vi "SNTP Light Initialization VI.vi"(8 "error in (no error)":errorcluster, 10 "Custom XML":string, 11 "Device Item Ref in":T1 format="%.0x") -> (0 "error out":errorcluster, 3 "Device Item Ref out":T1 format="%.0x")   [LabVIEW 2013, in "SNTP Light Custom Device Configuration.lvlib"]
uses:
  SNTP Light Custom Device Configuration.lvlib
  <vilib>/NI Veristand/Custom Device API/Custom Device Item Ref.ctl
  <vilib>/NI Veristand/Custom Device API/Custom Device Channel.ctl
  <vilib>/NI Veristand/Custom Device API/Custom Device Channel Type.ctl
  <vilib>/NI Veristand/Custom Device API/Set Item Property (String).vi
  <vilib>/NI Veristand/Custom Device API/Set Item Property (U16).vi
  <vilib>/NI Veristand/Custom Device API/Set Item Property (Double).vi
  <vilib>/NI Veristand/Custom Device API/Set Item Property (Boolean).vi
  <vilib>/NI Veristand/Custom Device API/Custom Device API.lvlib
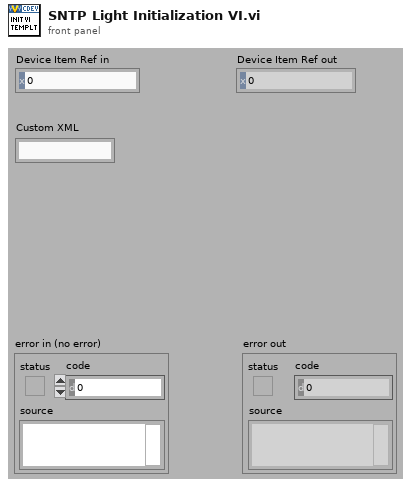
[diagram p1: front panel]
types:
  T1 = typedef "Custom Device API.lvlib/Custom Device Item Ref.ctl" = u64
  T2 = typedef "Custom Device API.lvlib/Custom Device Channel.ctl" = cluster{"Type":T3, "Units":string, "Default Value":dbl, "Faultable":bool, "Scalable":bool}
  T3 = typedef "Custom Device API.lvlib/Custom Device Channel Type.ctl" = enum16{"Input", "Output"}
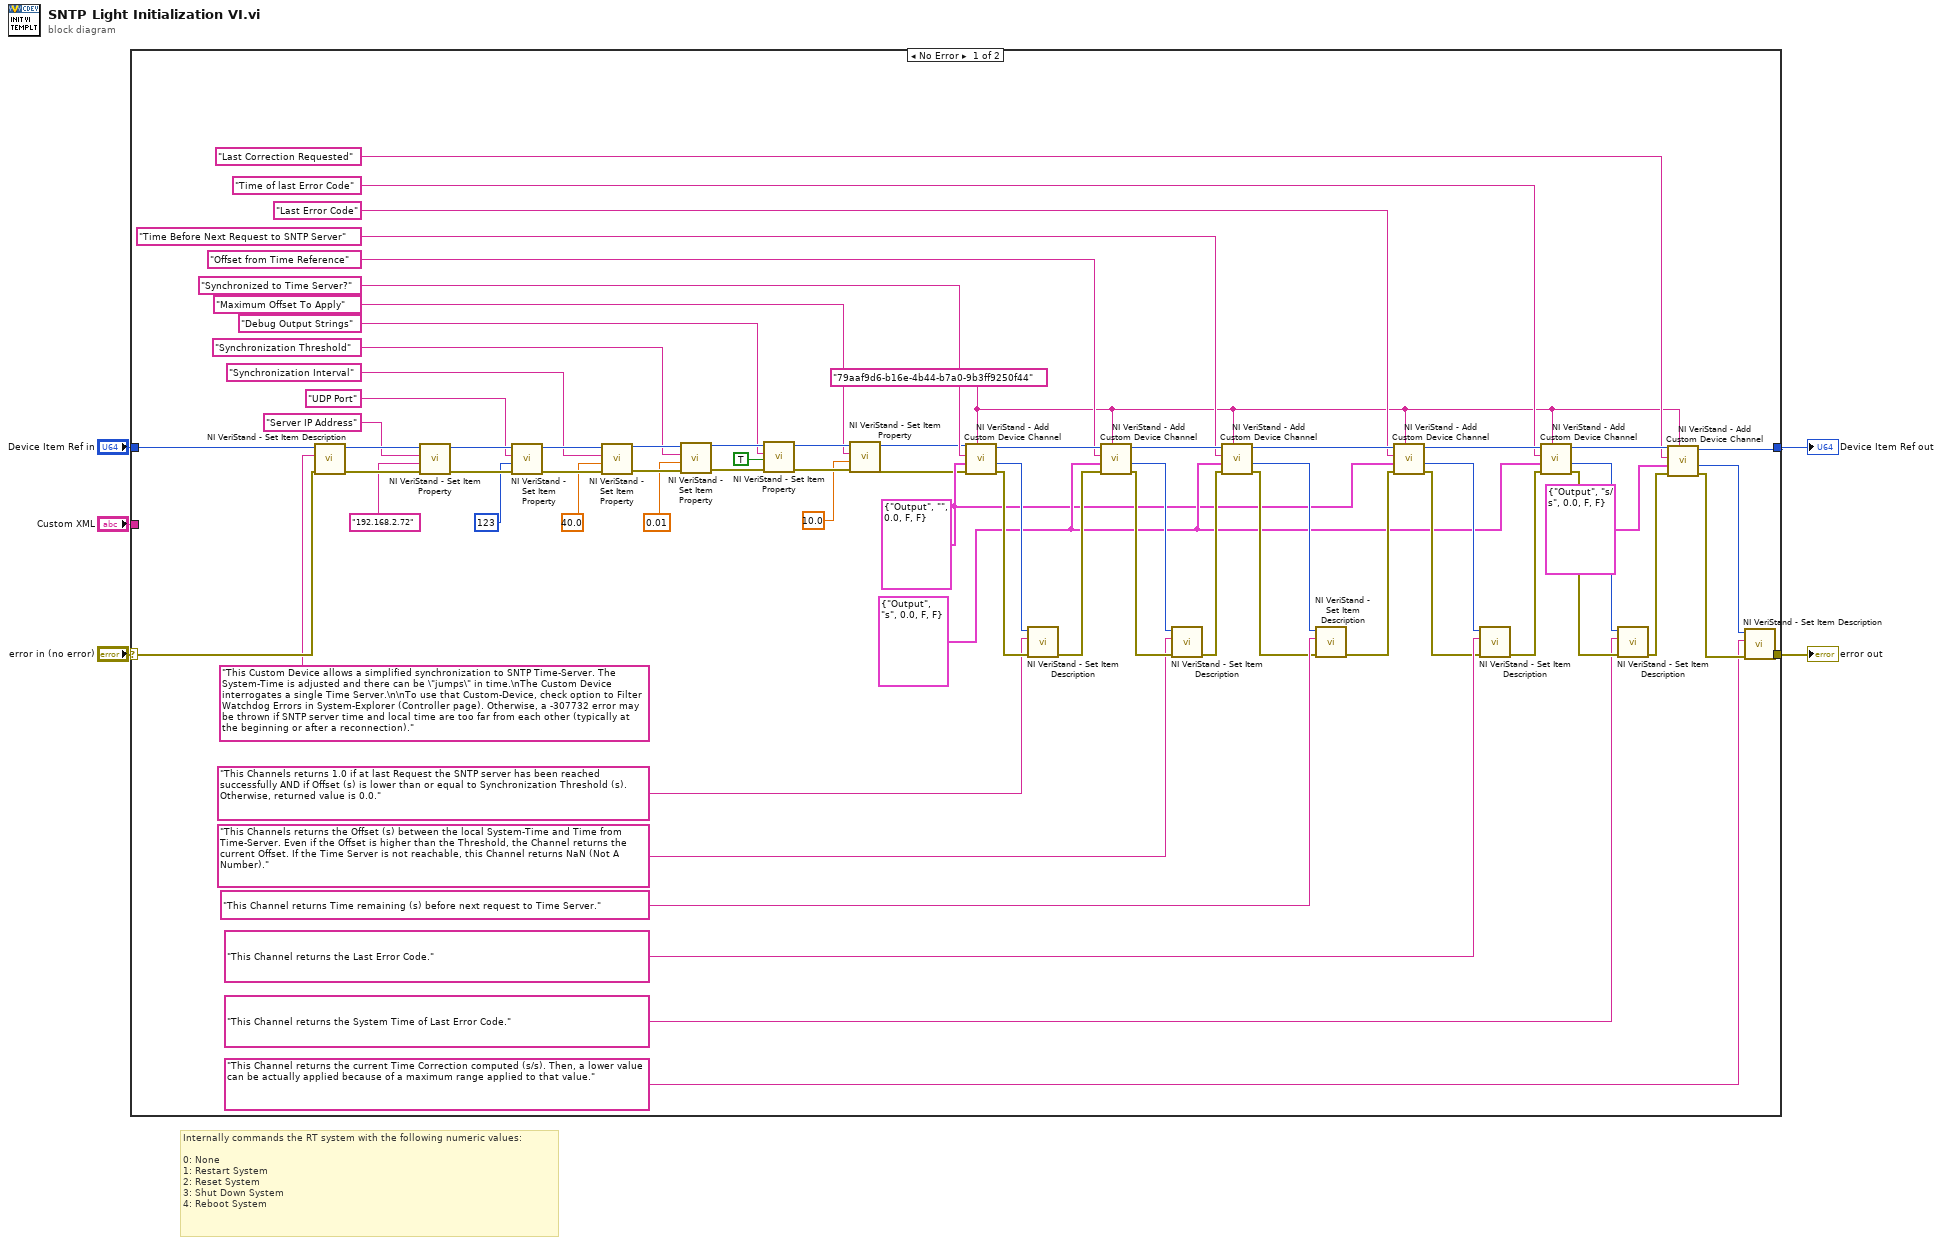
[diagram p0: block diagram]
diagram:
  # "Internally commands the RT system with the following numeric values:\n\n0: None\n1: Restart System\n2: Reset System\n3: Shut Down System\n4: Reboot System"
  n1 = case shown="No Error" "error in (no error)" {
    selector: "error in (no error)" -> [w73 w76]
    tunnel: [w6 w76] -> w5
    tunnel: [w7 w75] -> w3
    tunnel: "Device Item Ref in" -> [w74 w75]
    tunnel: "Custom XML" -> [_ _]
    frame No Error {
      w8 = "79aaf9d6-b16e-4b44-b7a0-9b3ff9250f44" ("GUID (Default Channel)")
      w19 = T2 {"Type"=enum."Output", "Units"="s", "Default Value"=0.0, "Faultable"=FALSE, "Scalable"=FALSE} ("Channel")
      w15 = T2 {"Type"=enum."Output", "Units"="", "Default Value"=0.0, "Faultable"=FALSE, "Scalable"=FALSE} ("Channel")
      n2 = call <vilib>:"NI VeriStand - Set Item Description.vi"("error in (no error)"=w73, "Description"="This Custom Device allows a simplified synchronization to SNTP Time-Server. The System-Time is adjusted and there can be \"jumps\" in time.\nThe Custom Device interrogates a single Time Server.\n\nTo use that Custom-Device, check option to Filter Watchdog Errors in System-Explorer (Controller page). Otherwise, a -307732 error may be thrown if SNTP server time and local time are too far from each other (typically at the beginning or after a reconnection).", "Item Ref in"=w74) -> ("error out"=w71:errorcluster, "Item Ref out"=w70:T1)  [unwired: 6 in, 1 out]
      n3 = call-poly <vilib>:"NI VeriStand - Set Item Property.vi"("error in (no error)"=w71, "Value"="192.168.2.72", "Property Name"="Server IP Address", "Item Ref in"=w70) -> ("error out"=w67:errorcluster, "Item Ref out"=w69:T1)  [unwired: 5 in, 1 out]
      n4 = call-poly <vilib>:"NI VeriStand - Set Item Property.vi"("error in (no error)"=w67, "Value"=u16 123, "Property Name"="UDP Port", "Item Ref in"=w69) -> ("error out"=w66:errorcluster, "Item Ref out"=w68:T1)  [unwired: 5 in, 1 out]
      n5 = call-poly <vilib>:"NI VeriStand - Set Item Property.vi"("error in (no error)"=w66, "Value"=40.0, "Property Name"="Synchronization Interval", "Item Ref in"=w68) -> ("error out"=w58:errorcluster, "Item Ref out"=w59:T1)  [unwired: 5 in, 1 out]
      n6 = call-poly <vilib>:"NI VeriStand - Set Item Property.vi"("error in (no error)"=w58, "Value"=0.01, "Property Name"="Synchronization Threshold", "Item Ref in"=w59) -> ("error out"=w30:errorcluster, "Item Ref out"=w31:T1)  [unwired: 5 in, 1 out]
      n7 = call-poly <vilib>:"NI VeriStand - Set Item Property.vi"("error in (no error)"=w30, "Value"=TRUE, "Property Name"="Debug Output Strings", "Item Ref in"=w31) -> ("error out"=w11:errorcluster, "Item Ref out"=w14:T1)  [unwired: 5 in, 1 out]
      n8 = call-poly <vilib>:"NI VeriStand - Set Item Property.vi"("error in (no error)"=w11, "Value"=10.0, "Property Name"="Maximum Offset To Apply", "Item Ref in"=w14) -> ("error out"=w12:errorcluster, "Item Ref out"=w13:T1)  [unwired: 5 in, 1 out]
      n9 = call <vilib>:"NI VeriStand - Add Custom Device Channel.vi"("GUID (Default Channel)"=w8, "error in (no error)"=w12, "Channel"=w15, "Channel Name"="Synchronized to Time Server?", "Parent Ref in"=w13) -> ("error out"=w54:errorcluster, "Channel Ref"=w53:T1, "Parent Ref out"=w51:T1)  [unwired: 3 in, 1 out]
      n10 = call <vilib>:"NI VeriStand - Set Item Description.vi"("error in (no error)"=w54, "Description"="This Channels returns 1.0 if at last Request the SNTP server has been reached successfully AND if Offset (s) is lower than or equal to Synchronization Threshold (s). Otherwise, returned value is 0.0.", "Item Ref in"=w53) -> ("error out"=w50:errorcluster)  [unwired: 6 in, 2 out]
      n11 = call <vilib>:"NI VeriStand - Add Custom Device Channel.vi"("GUID (Default Channel)"=w8, "error in (no error)"=w50, "Channel"=w19, "Channel Name"="Offset from Time Reference", "Parent Ref in"=w51) -> ("error out"=w48:errorcluster, "Channel Ref"=w47:T1, "Parent Ref out"=w46:T1)  [unwired: 3 in, 1 out]
      n12 = call <vilib>:"NI VeriStand - Set Item Description.vi"("error in (no error)"=w48, "Description"="This Channels returns the Offset (s) between the local System-Time and Time from Time-Server. Even if the Offset is higher than the Threshold, the Channel returns the current Offset. If the Time Server is not reachable, this Channel returns NaN (Not A Number).", "Item Ref in"=w47) -> ("error out"=w45:errorcluster)  [unwired: 6 in, 2 out]
      n13 = call <vilib>:"NI VeriStand - Add Custom Device Channel.vi"("GUID (Default Channel)"=w8, "error in (no error)"=w45, "Channel"=w19, "Channel Name"="Time Before Next Request to SNTP Server", "Parent Ref in"=w46) -> ("error out"=w42:errorcluster, "Channel Ref"=w41:T1, "Parent Ref out"=w39:T1)  [unwired: 3 in, 1 out]
      n14 = call <vilib>:"NI VeriStand - Set Item Description.vi"("error in (no error)"=w42, "Description"="This Channel returns Time remaining (s) before next request to Time Server.", "Item Ref in"=w41) -> ("error out"=w40:errorcluster)  [unwired: 6 in, 2 out]
      n15 = call <vilib>:"NI VeriStand - Add Custom Device Channel.vi"("GUID (Default Channel)"=w8, "error in (no error)"=w40, "Channel"=w15, "Channel Name"="Last Error Code", "Parent Ref in"=w39) -> ("error out"=w36:errorcluster, "Channel Ref"=w32:T1, "Parent Ref out"=w34:T1)  [unwired: 3 in, 1 out]
      n16 = call <vilib>:"NI VeriStand - Set Item Description.vi"("error in (no error)"=w36, "Description"="This Channel returns the Last Error Code.", "Item Ref in"=w32) -> ("error out"=w35:errorcluster)  [unwired: 6 in, 2 out]
      n17 = call <vilib>:"NI VeriStand - Add Custom Device Channel.vi"("GUID (Default Channel)"=w8, "error in (no error)"=w35, "Channel"=w19, "Channel Name"="Time of last Error Code", "Parent Ref in"=w34) -> ("error out"=w26:errorcluster, "Channel Ref"=w25:T1, "Parent Ref out"=w21:T1)  [unwired: 3 in, 1 out]
      n18 = call <vilib>:"NI VeriStand - Set Item Description.vi"("error in (no error)"=w26, "Description"="This Channel returns the System Time of Last Error Code.", "Item Ref in"=w25) -> ("error out"=w20:errorcluster)  [unwired: 6 in, 2 out]
      n19 = call <vilib>:"NI VeriStand - Add Custom Device Channel.vi"("GUID (Default Channel)"=w8, "error in (no error)"=w20, "Channel"=T2 {"Type"=enum."Output", "Units"="s/s", "Default Value"=0.0, "Faultable"=FALSE, "Scalable"=FALSE}, "Channel Name"="Last Correction Requested", "Parent Ref in"=w21) -> ("error out"=w22:errorcluster, "Channel Ref"=w23:T1, "Parent Ref out"=w7:T1)  [unwired: 3 in, 1 out]
      n20 = call <vilib>:"NI VeriStand - Set Item Description.vi"("error in (no error)"=w22, "Description"="This Channel returns the current Time Correction computed (s/s). Then, a lower value can be actually applied because of a maximum range applied to that value.", "Item Ref in"=w23) -> ("error out"=w6:errorcluster)  [unwired: 6 in, 2 out]
    }
    frame Error {
    }
  }
  "error out" <- w5
  "Device Item Ref out" <- w3
